vi "Configure Dialog.vi"(7 "Data in":path, 11 "Static Path Selector in":refnum<class "MGI Static Path Selector.lvclass">) -> (2 "Changed?":bool, 3 "Static Path Selector out":refnum<class "MGI Static Path Selector.lvclass">, 5 "Data out":path)   [LabVIEW 2020, in "MGI Static Path Selector.lvclass"]
uses:
  <userlib>/_MGI/User Interface/Path Selector XControl/Class Hierarchy/Static File Selector/MGI Static Path Selector.lvclass
  <userlib>/_MGI/User Interface/Path Selector XControl/Control Style Enum.ctl
  <userlib>/_MGI/User Interface/Path Selector XControl/Class Hierarchy/Static File Selector/MGI Static Path Selector.lvclass/MGI Static Path Selector.ctl
  <userlib>/_MGI/User Interface/Path Selector XControl/MGI Path Selector.xctl
panel:
  in  "Control Style":T1
  in  "Filter":string(combo) caption="Filter: Type in desired filter or select existing option below:"
  in  "Browse Option":bool
  in  "Explore Option":bool
  in  "Allow New":bool
  in  "Recursive List":bool
  in  "Path":path
  in  "Done":bool
  # "This dialog allows configuration of the File Selector.\nThe file selector is a combo box that shows files from a directory and allows the user to select a file.    The directory containing the files (file directory) is typically the folder containing the file last selected by the user.  The File Selector remembers which file is selected by the user by saving this information to a file."
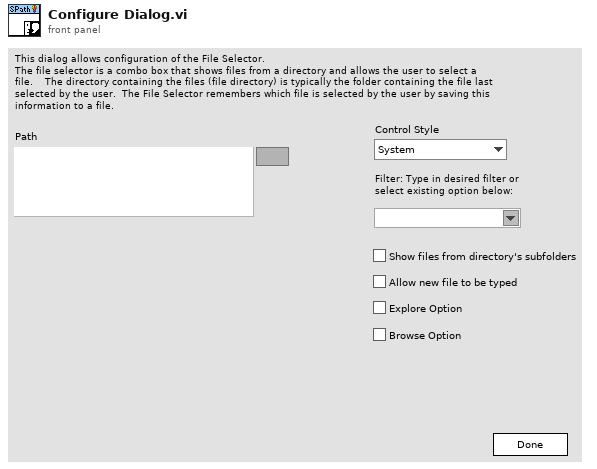
[diagram p1: front panel]
types:
  T1 = typedef "MGI Path Selector.xctl/Control Style Enum.ctl" = enum16{"System", "Modern", "Classic", "Silver"}
  T2 = enum16{"Left Button", "Center Button", "Right Button", "Window Close"}
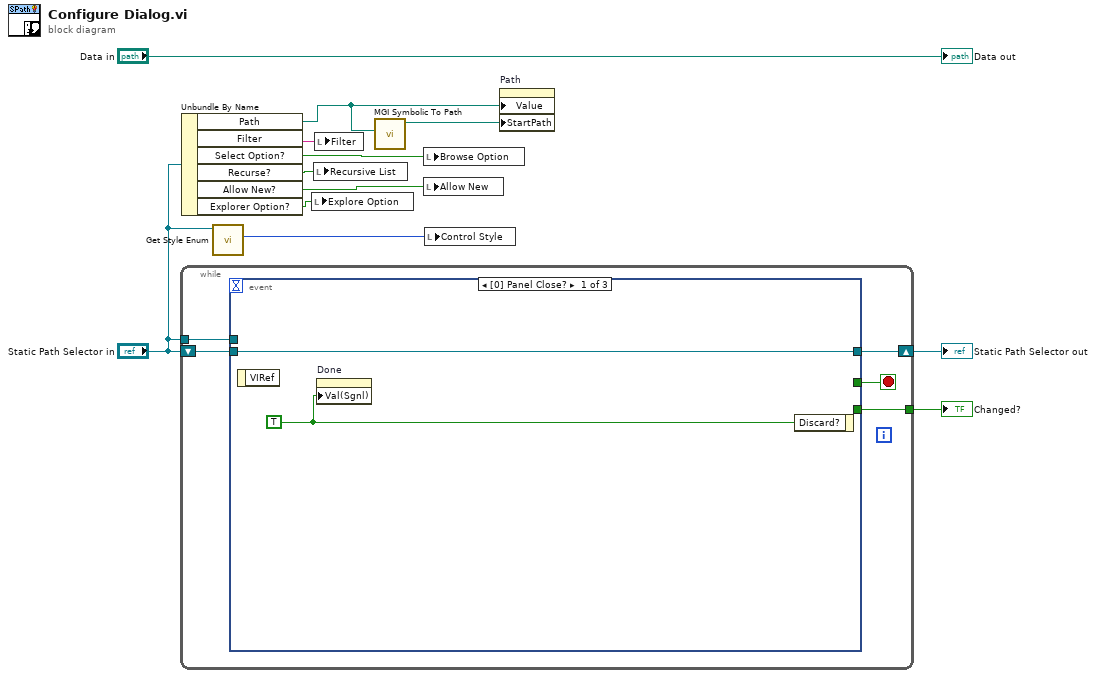
[diagram p0: block diagram]
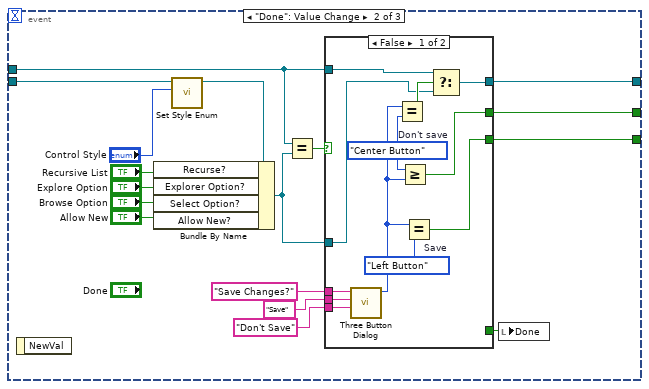
[diagram p2: hidden frame]
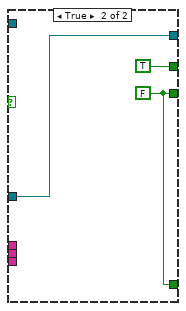
[diagram p3: hidden frame]
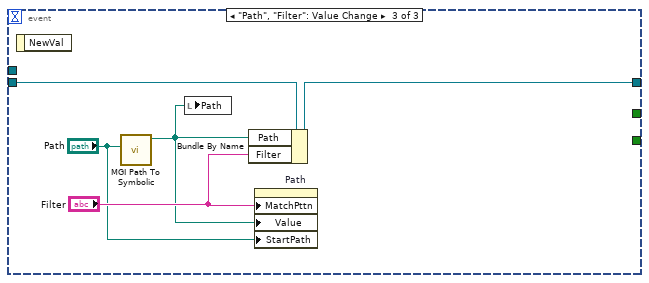
[diagram p4: hidden frame]
diagram:
  n1 = while {
    shift-right: [w13] -> w9
    shift-left: "Static Path Selector in" -> [w17]
    tunnel: "Static Path Selector in" -> [w16]
    tunnel: [w14] -> w8
    stop <- w15 stop-if-true
    n2 = event shown="[0] Panel Close?" {
      selector: _ -> [_ _ _]
      dyn-events: _ -> [_ _ _]
      timeout: _ -> [_ _ _]
      tunnel: w17 -> [w19 w22 w56]
      tunnel: w16 -> [_ w31 _]
      tunnel: [_ w26 _] -> w15
      tunnel: [_ w25 _] -> w14
      tunnel: [w19 w27 w55] -> w13
      event Panel Close? {
        w18 = TRUE ("Discard?")
        n3 = event-data() -> ()  [unwired: 1 in, 1 out]
        n4 = property on="Done" class="Bool (strict)"("Val(Sgnl)"=w18) -> ()  [unwired: 2 in, 2 out]
        n5 = event-data("Discard?"=w18) -> ()  [unwired: 1 in, 1 out]
      }
      event "Done": Value Change {
        n6 = event-data() -> ()  [unwired: 1 in, 1 out]
        n7 = call-dynamic "Set Style Enum.vi"("Control Style"="Control Style", "Path Selector in"=w22) -> ("Path Selector out"=w21:refnum<class "MGI Static Path Selector.lvclass">)  [unwired: 9 in]
        n8 = Bundle By Name(cluster=w21, "Recurse?"="Recursive List", "Explorer Option?"="Explore Option", "Select Option?"="Browse Option", "Allow New?"="Allow New") -> (w23:refnum<class "MGI Static Path Selector.lvclass">)
        n9 = Equal?(x=w31, y=w23) -> (x = y?=w32:bool)
        n10 = case shown="False" w32 {
          tunnel: w31 -> [w42 _]
          tunnel: "Save Changes?" ("message") -> [w48 _]
          tunnel: "Save" ("Left Button Text (\"Yes\")") -> [w47 _]
          tunnel: "Don't Save" ("Center Button Text (\"No\")") -> [w46 _]
          tunnel: [w41 w49] -> w27
          tunnel: [w45 TRUE] -> w26
          tunnel: [w38 w50] -> w25
          tunnel: [_ w50] -> w24
          tunnel: w23 -> [w37 w49]
          frame False {
            w39 = T2."Left Button"  # Save
            w44 = T2."Center Button"  # Don't save
            n11 = call <vilib>:"Three Button Dialog.vi"("Center Button Text (\"No\")"=w46, "Left Button Text (\"Yes\")"=w47, "message"=w48) -> ("Which Button?"=w40:T2)  [unwired: 8 in]
            n12 = Equal?(x=w40, y=w44) -> (x = y?=w43:bool)
            n13 = Greater Or Equal?(x=w44, y=w40) -> (x >= y?=w45:bool)
            n14 = Equal?(x=w40, y=w39) -> (x = y?=w38:bool)
            n15 = Select(t=w42, s=w43, f=w37) -> (s? t:f=w41:refnum<class "MGI Static Path Selector.lvclass">)
          }
          frame True {
            w50 = FALSE
          }
        }
        n16 = local write "Done"(w24) -> ()
      }
      event "Path", "Filter": Value Change {
        n17 = event-data() -> ()  [unwired: 1 in, 1 out]
        n18 = call <userlib>:"MGI Path To Symbolic.vi"("Path"="Path") -> ("Symbolic Path"=w52:path)  [unwired: 8 in, 2 out]
        n19 = local write "Path"(w52) -> ()
        n20 = Bundle By Name(cluster=w56, "Path"=w52, "Filter"="Filter") -> (w55:refnum<class "MGI Static Path Selector.lvclass">)
        n21 = property on="Path" class="Path"("MatchPttn"="Filter", "Value"=w52, "StartPath"="Path") -> ()  [unwired: 2 in, 2 out]
      }
    }
  }
  "Changed?" <- w8
  "Static Path Selector out" <- w9
  n22 = Unbundle By Name("Static Path Selector in") -> ("Path"=w2:path, "Filter"=w10:string, "Select Option?"=w7:bool, "Recurse?"=w6:bool, "Allow New?"=w5:bool, "Explorer Option?"=w11:bool)
  n23 = call-dynamic "Get Style Enum.vi"("Path Selector in"="Static Path Selector in") -> ("Control Style"=w3:T1)  [unwired: 10 in]
  n24 = local write "Explore Option"(w11) -> ()
  n25 = local write "Recursive List"(w6) -> ()
  n26 = local write "Filter"(w10) -> ()
  n27 = call <userlib>:"MGI Symbolic To Path.vi"("Symbolic Path"=w2) -> ("Path"=w1:path)  [unwired: 8 in, 2 out]
  n28 = local write "Browse Option"(w7) -> ()
  n29 = local write "Allow New"(w5) -> ()
  n30 = local write "Control Style"(w3) -> ()
  n31 = property on="Path" class="Path"("Value"=w2, "StartPath"=w1) -> ()  [unwired: 2 in, 2 out]
  "Data out" <- "Data in"
